vi "Build Installed Folder Paths.vi"() -> (2 "Application Folder Path":path, 3 "Data Folder Path":path)   [LabVIEW 2021, in "CANOpen Addon System Explorer.lvlib"]
uses:
  CANOpen Addon System Explorer.lvlib
  <vilib>/Utility/sysdir.llb/System Directory Type.ctl
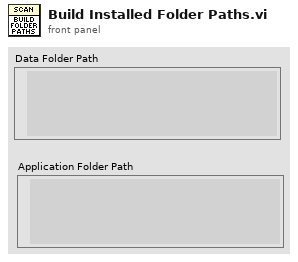
[diagram p1: front panel]
types:
  T1 = typedef "System Directory Type.ctl" = i32
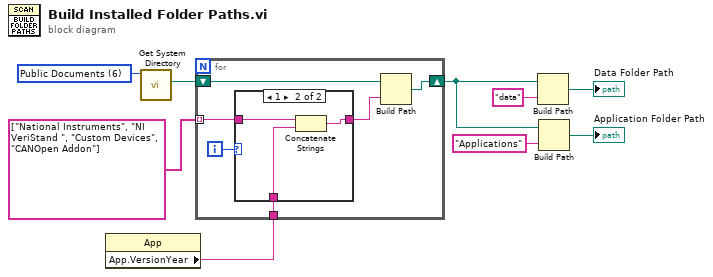
[diagram p0: block diagram]
diagram:
  w9 = T1 6 items=["User Home"=0, "User Desktop"=1, "User Documents"=2, "User Application Data"=3, "User Preferences"=4, "User Temporary"=5, "Public Documents"=6, "Public Application Data"=7, "Public Preferences"=8, "Public Cache"=13, "System Core Libraries"=9, "System Installed Libraries"=10, "Application Files"=11, "Boot Volume Root"=12] ("system directory type")
  n1 = property class="App"() -> ("App.VersionYear"=w6:string)  [unwired: 2 in, 2 out]
  n2 = call <vilib>:"Get System Directory.vi"("system directory type"=w9) -> ("system directory"=w8:path)  [unwired: 10 in]
  n3 = for {
    shift-right: [w14] -> w4
    shift-left: w8 -> [w15]
    tunnel: string[] ["National Instruments", "NI VeriStand ", "Custom Devices", "CANOpen Addon"] -> [w11] mode=indexing
    tunnel: w6 -> [w10]
    i -> [w13]
    n4 = case shown="1" w13 {
      tunnel: [w16 w18] -> w12
      tunnel: w11 -> [w16 w19]
      tunnel: w10 -> [_ w17]
      frame Default {
      }
      frame 1 {
        n5 = Concatenate Strings(w19, w17) -> (w18:string)
      }
    }
    n6 = Build Path(base path=w15, name or relative path=w12) -> (appended path=w14:path)
  }
  n7 = Build Path(base path=w4, name or relative path="data") -> (appended path=→"Data Folder Path":path)
  n8 = Build Path(base path=w4, name or relative path="Applications") -> (appended path=→"Application Folder Path":path)
